vi "Write Formats.vi"(8 "error in (no error)":errorcluster, 10 "Formats":T1[](array[typedef]), 11 "ZXing Options in":refnum<class "ZXing Options.lvclass">) -> (0 "error out":errorcluster, 3 "ZXing Options out":refnum<class "ZXing Options.lvclass">)   [LabVIEW 2020, in "feature_detection.lvlib" / "ZXing Options.lvclass"]
uses:
  ZXing Options.lvclass
  ZXing Options.lvclass/ZXing Options.ctl
  Format.ctl
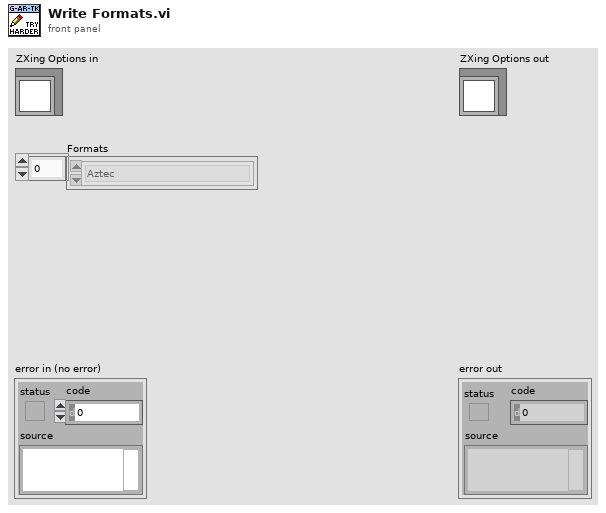
[diagram p1: front panel]
types:
  T1 = typedef "feature_detection.lvlib/ZXing Options.lvclass/Format.ctl" = enum8{"Aztec", "Codabar", "Code 39", "Code 93", "Code 128", "Data Bar", "Data Bar Expanded", "Data Matrix", "EAN 8", "EAN 13", "ITF", "Maxi Code", "PDF417", "QR Code", "UPCA", "UPCE", "Micro QR Code", "RM QR Code", "DX Film Edge", "Data Bar Limited"}
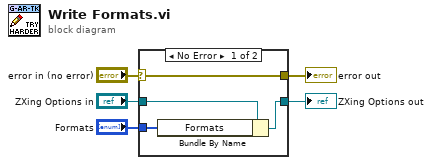
[diagram p0: block diagram]
diagram:
  n1 = case shown="No Error" "error in (no error)" {
    selector: "error in (no error)" -> [w9 w10]
    tunnel: [w9 w10] -> w4
    tunnel: [w6 w11] -> w2
    tunnel: "ZXing Options in" -> [w8 w11]
    tunnel: "Formats" -> [w7 _]
    frame No Error {
      n2 = Bundle By Name(cluster=w8, "Formats"=w7) -> (w6:refnum<class "ZXing Options.lvclass">)
    }
    frame Error {
    }
  }
  "error out" <- w4
  "ZXing Options out" <- w2
